vi "Area_Check2Total_Main Function.vi"(11 "img in":T3) -> (0 "error out":errorcluster, 1 "AreaDataOut":T2(array[cluster]) {"AreaDataOut"."Rectangle"."Rotation" format="%.2f"; "AreaDataOut"."Rectangle"."Left" scale=0.0..1024.0; "AreaDataOut"."Rectangle"."Right" scale=0.0..1024.0}, 2 "Array":dbl[](array[numeric]), 3 "Iimg out":T3)   [LabVIEW 2019]
uses:
  <vilib>/vision/Image Controls.llb/IMAQ Image.ctl
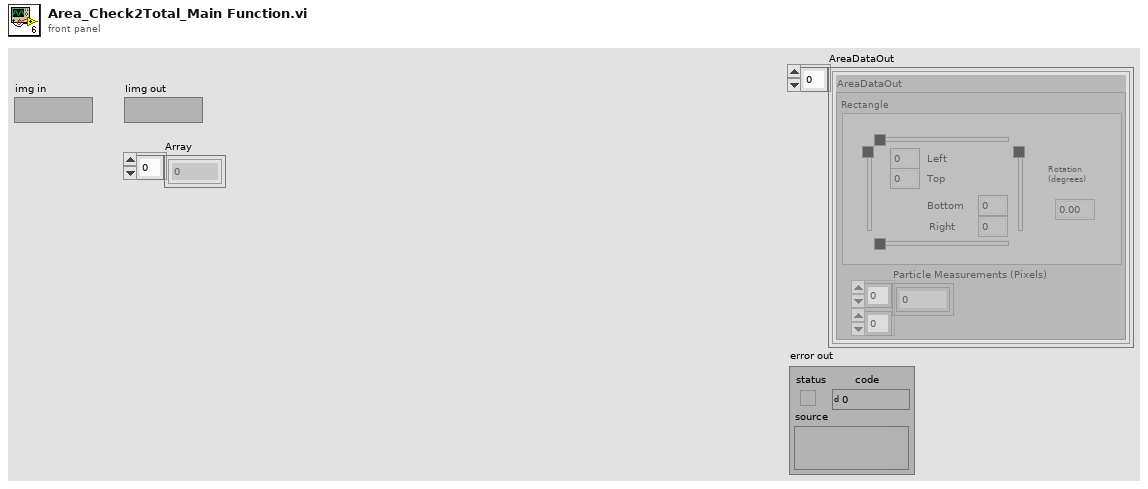
[diagram p1: front panel]
types:
  T1 = typedef "IMAQ Rectangle" = cluster{"Left":i32, "Top":i32, "Right":i32, "Bottom":i32, "Rotation":dbl}
  T2 = cluster{"AreaDataOut":cluster{"Rectangle":T1, "Particle Measurements (Pixels)":dbl[][]}}[]
  T3 = typedef "IMAQ Image.ctl" = refnum<image>
  T4 = cluster{"AreaDataOut":cluster{"Rectangle":T1, "Particle Measurements (Pixels)":dbl[][]}}
  T5 = cluster{"Rectangle":T1, "Particle Measurements (Pixels)":dbl[][]}
  T6 = cluster{dbl, dbl, "X Resolution":i32, "Y Resolution":i32, dbl}
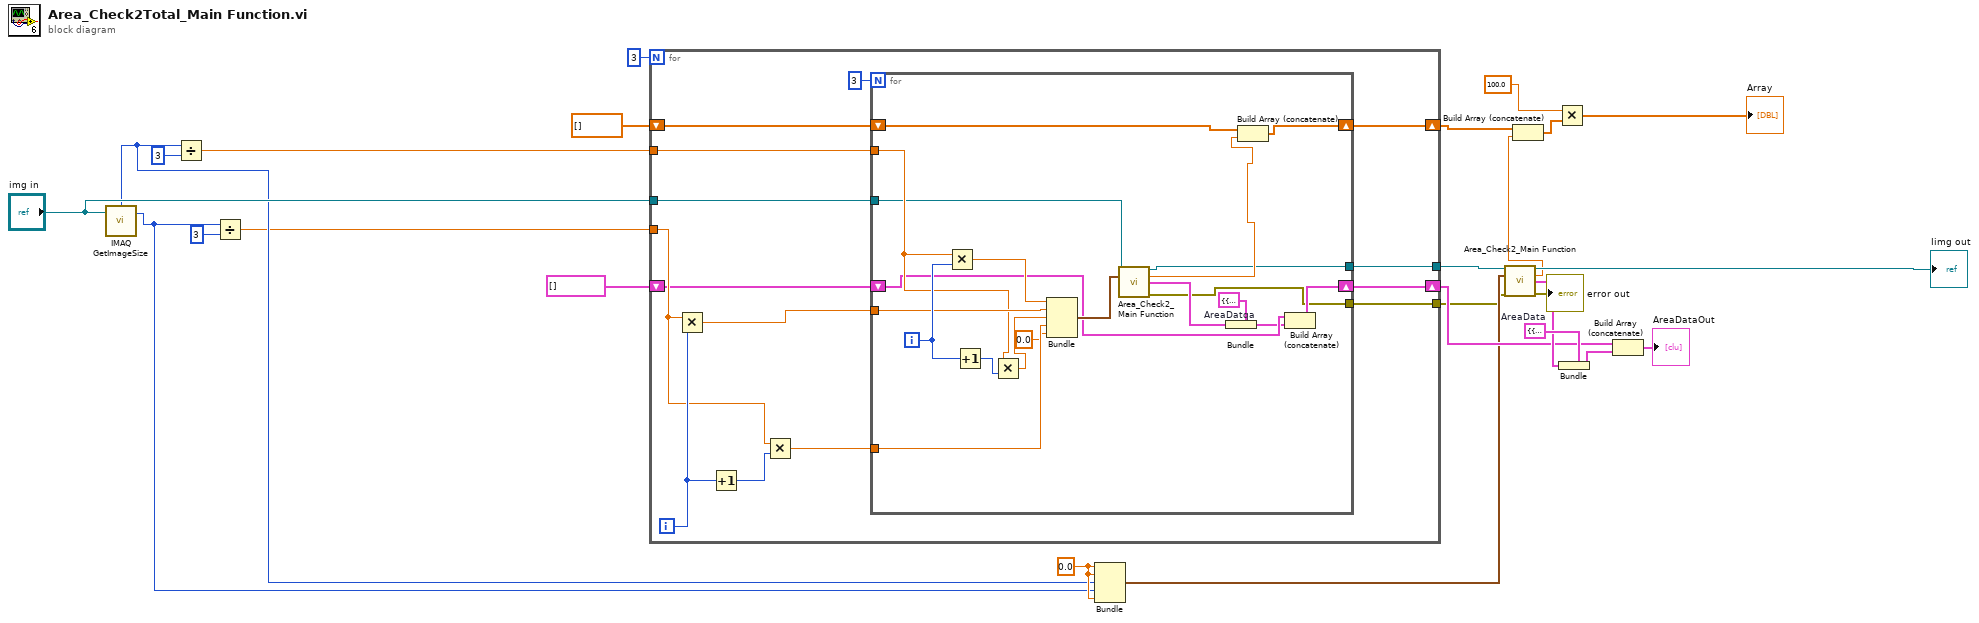
[diagram p0: block diagram]
diagram:
  w25 = T4 {"AreaDataOut"={"Rectangle"={"Left"=0, "Top"=0, "Right"=0, "Bottom"=0, "Rotation"=0.0}, "Particle Measurements (Pixels)"=[]}}  # AreaData
  w13 = 0.0
  n1 = call "IMAQ GetImageSize"("Image"="img in") -> ("Y Resolution"=w12:i32, "X Resolution"=w11:i32)  [unwired: 3 in, 1 out]
  n2 = Divide(x=w11, y=3) -> (x/y=w6:dbl)
  n3 = Divide(x=w12, y=3) -> (x/y=w7:dbl)
  n4 = for {
    N: 3 -> [_]
    tunnel: w6 -> [w40]
    tunnel: w7 -> [w37]
    tunnel: "img in" -> [w34]
    shift-right: [w31] -> w15
    shift-left: dbl[] [] -> [w32]
    tunnel: [w30] -> w10
    shift-right: [w29] -> w22
    shift-left: T2 [] -> [w28]
    tunnel: [w27] -> w2
    i -> [w39]
    n5 = Multiply(x=w37, y=w39) -> (x*y=w36:dbl)
    n6 = Increment(x=w39) -> (x+1=w38:i32)
    n7 = Multiply(x=w37, y=w38) -> (x*y=w35:dbl)
    n8 = for {
      N: 3 -> [_]
      tunnel: w40 -> [w56]
      tunnel: w36 -> [w57]
      tunnel: w35 -> [w55]
      tunnel: w34 -> [w52]
      shift-right: [w49] -> w31
      shift-left: w32 -> [w50]
      tunnel: [w47] -> w30
      shift-right: [w45] -> w29
      shift-left: w28 -> [w44]
      tunnel: [w41] -> w27
      i -> [w60]
      w42 = T4 {"AreaDataOut"={"Rectangle"={"Left"=0, "Top"=0, "Right"=0, "Bottom"=0, "Rotation"=0.0}, "Particle Measurements (Pixels)"=[]}}  # AreaDatqa
      n9 = Multiply(x=w56, y=w60) -> (x*y=w58:dbl)
      n10 = Increment(x=w60) -> (x+1=w59:i32)
      n11 = Multiply(x=w56, y=w59) -> (x*y=w51:dbl)
      n12 = Bundle(w58, w57, w51, w55, 0.0) -> (w53:cluster{dbl, dbl, dbl, dbl, dbl})  [unwired: 1 in]
      n13 = call "Area_Check2_Main Function.vi"("Image Src"=w52, "Rectangle"=w53) -> ("Image Out"=w47:T3, "%"=w48:dbl, "AreaDataOut"=w46:T5, "error out"=w41:errorcluster)  [unwired: 10 in]
      n14 = Bundle(cluster=w42, "AreaDataOut"=w46) -> (w43:T4)
      n15 = Build Array (concatenate)(w50, w48) -> (w49:dbl[])
      n16 = Build Array (concatenate)(w44, w43) -> (w45:T2)
    }
  }
  n17 = Bundle(w13, w13, "X Resolution"=w11, "Y Resolution"=w12, w13) -> (w14:T6)  [unwired: 1 in]
  n18 = call "Area_Check2_Main Function.vi"("Image Src"=w10, "Rectangle"=w14, "error in"=w2) -> ("Image Out"=→"Iimg out":T3, "%"=w16:dbl, "AreaDataOut"=w24:T5, "error out"=→"error out":errorcluster)  [unwired: 9 in]
  n19 = Build Array (concatenate)(w15, w16) -> (w17:dbl[])
  n20 = Multiply(x=100.0, y=w17) -> (x*y=→"Array":dbl[])
  n21 = Bundle(cluster=w25, "AreaDataOut"=w24) -> (w23:T4)
  n22 = Build Array (concatenate)(w22, w23) -> (→"AreaDataOut":T2)
